vi "Adjusted_Mutual_Info_Score.vi"(8 "error in":errorcluster caption="entrée d'erreur", 9 "labels_pred":string[][](array[string]), 10 "labels_true":string[][](array[string]), 11 "adjusted_mutual_info_score":cluster{"average_method":string}={"average_method"="arithmetic"}) -> (0 "error out":errorcluster caption="sortie d'erreur", 3 "Score":string)   [LabVIEW 2020]
doc: "Adjusted Mutual Information between two clusterings.\n\nAdjusted Mutual Information (AMI) is an adjustment of the Mutual Information (MI) score to account for chance. It accounts for the fact that the MI is generally higher for two clusterings with a larger number of clusters, regardless of whether there is actually more information shared. For two clusterings U and V , the AMI is given as :\n\nAMI(U, V) = [MI(U, V) - E(MI(U, V))] / [avg(H(U), H(V)) - E(MI(U, V))]\n\nThis metric is independent of the absolute values of the labels: a permutation of the class or cluster label values won’t change the score value in any way.\n\nThis metric is furthermore symmetric: switching label_true with label_pred will return the same score value. This can be useful to measure the agreement of two independent label assignments strategies on the same dataset when the real ground truth is not known.\n\nBe mindful that this function is an order of magnitude slower than other metrics, such as the Adjusted Rand Index.\n\n\nParameters : \n\n- labels_true : int array, shape = [n_samples]\nA clustering of the data into disjoint subsets.\n\n- labels_pred : int array-like of shape (n_samples,)\nA clustering of the data into disjoint subsets.\n\n- average_method : string, optional (default: ‘arithmetic’)\nHow to compute the normalizer in the denominator. Possible options are ‘min’, ‘geometric’, ‘arithmetic’, and ‘max’.\n\nReturns : \n\n- ami : float (upperlimited by 1.0)\nThe AMI returns a value of 1 when the two partitions are identical (ie perfectly matched). Random partitions (independent labellings) have an expected AMI around 0 on average hence can be negative."
uses:
  Adjusted_Mutual_Info_Score.lvclass
panel:
  out "Adjusted_Mutual_Info_Score.lvclass":refnum<class "Adjusted_Mutual_Info_Score.lvclass">
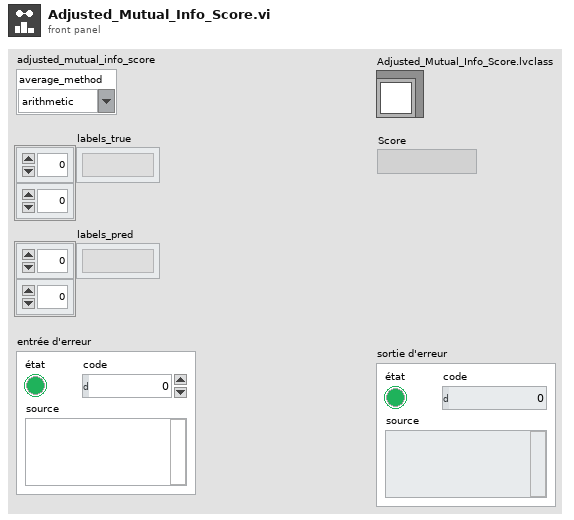
[diagram p1: front panel]
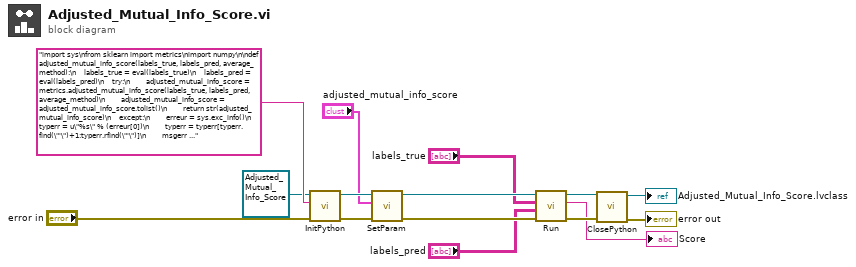
[diagram p0: block diagram]
diagram:
  n1 = call-dynamic "InitPython.vi"("error in (no error)"="error in", "Python Instruction"="import sys\nfrom sklearn import metrics\nimport numpy\n\ndef adjusted_mutual_info_score(labels_true, labels_pred, average_method):\n    labels_true = eval(labels_true)\n    labels_pred = eval(labels_pred)\n    try:\n        adjusted_mutual_info_score = metrics.adjusted_mutual_info_score(labels_true, labels_pred, average_method)\n        adjusted_mutual_info_score = adjusted_mutual_info_score.tolist()\n        return str(adjusted_mutual_info_score)\n    except:\n        erreur = sys.exc_info()\n        typerr = u\"%s\" % (erreur[0])\n        typerr = typerr[typerr.find(\"'\")+1:typerr.rfind(\"'\")]\n        msgerr = u\"%s\" % (erreur[1])\n        message = str('/!\\\\ {0} : {1}'. format(typerr,msgerr))\n        return message", "Scikit-learn en entrée"=refnum<class "Adjusted_Mutual_Info_Score.lvclass"> refnum ("Adjusted_Mutual_Info_Score.lvclass")) -> ("error out"=w10:errorcluster, "Scikit-learn en sortie"=w11:refnum<class "Adjusted_Mutual_Info_Score.lvclass">)  [unwired: 7 in]
  n2 = call-dynamic "SetParam.vi"("error in (no error)"=w10, "adjusted_mutual_info_score"="adjusted_mutual_info_score", "Adjusted_Mutual_Info_Score.lvclass"=w11) -> ("error out"=w7:errorcluster, "Adjusted_Mutual_Info_Score.lvclass"=w8:refnum<class "Adjusted_Mutual_Info_Score.lvclass">)  [unwired: 7 in]
  n3 = call-dynamic "Run.vi"("error in (no error)"=w7, "labels_pred"="labels_pred", "labels_true"="labels_true", "Adjusted_Mutual_Info_Score.lvclass"=w8) -> ("error out"=w5:errorcluster, "String Data"=→"Score":string, "Adjusted_Mutual_Info_Score.lvclass"=w6:refnum<class "Adjusted_Mutual_Info_Score.lvclass">)  [unwired: 5 in]
  n4 = call-dynamic "ClosePython.vi"("error in (no error)"=w5, "Scikit-learn en entrée"=w6) -> ("error out"=→"error out":errorcluster, "Scikit-learn en sortie"=→"Adjusted_Mutual_Info_Score.lvclass":refnum<class "Adjusted_Mutual_Info_Score.lvclass">)  [unwired: 8 in]
